vi "Execute Tests.vi"(8 "error in (no error)":errorcluster, 10 "Tests":string[](array[string]), 11 "Execution UI In":refnum<class "Execution UI.lvclass">) -> (0 "error out":errorcluster, 3 "Execution UI Out":refnum<class "Execution UI.lvclass">)   [LabVIEW 2020, in "Execution UI.lvclass"]
uses:
  Execution UI.lvclass
  TypeDefs/Execution State.ctl
  Result Model by Reference/Result Model by Reference.lvclass
  API/LUnit Test Suite/LUnit Test Suite.lvclass
  Support/Filters/Static Filter/Static Filter.lvclass
  Support/Filters/Dashed Filter/Dashed Filter.lvclass
  Support/Filters/Filter/Filter.lvclass
  Framework/Plugin/Plugin.lvclass
  Framework/Test Runner/Test Runner.lvclass
  C:/git/astemes-lunit/source/Core/Runnable/Runnable.lvclass
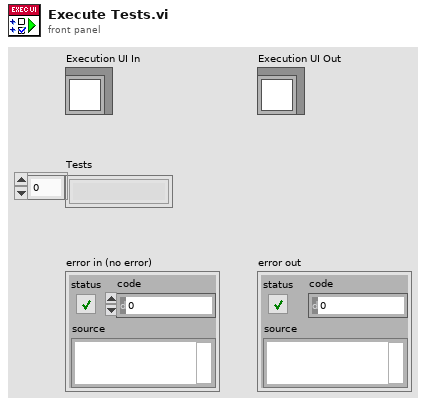
[diagram p1: front panel]
types:
  T1 = typedef "Execution UI.lvclass/Execution State.ctl" = enum16{"Idle", "Running"}
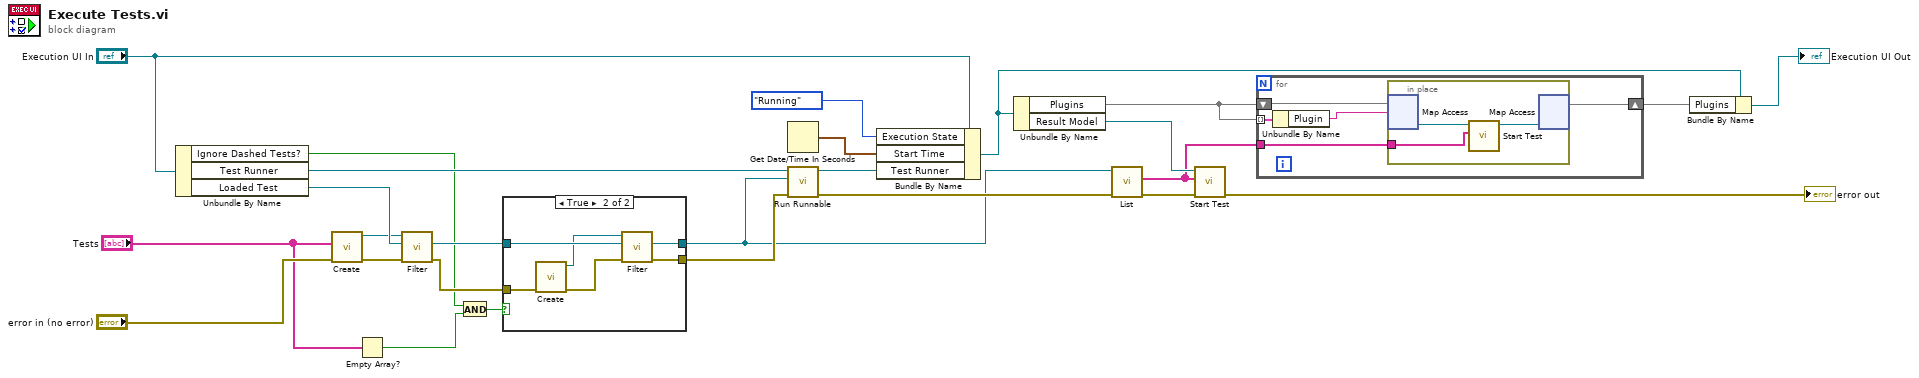
[diagram p0: block diagram]
diagram:
  n1 = Unbundle By Name("Execution UI In") -> ("Ignore Dashed Tests?"=w4:bool, "Test Runner"=w26:refnum<class "Test Runner.lvclass">, "Loaded Test"=w12:refnum<class "LUnit Test Suite.lvclass">)
  n2 = call "Create.vi"("error in (no error)"="error in (no error)", "Tests"="Tests") -> ("error out"=w9:errorcluster, "Static Filter"=w10:refnum<class "Filter.lvclass">)  [unwired: 8 in]
  n3 = Empty Array?(array="Tests") -> (empty?=w1:bool)
  n4 = call-dynamic "Filter.vi"("error in (no error)"=w9, "Test Suite"=w12, "Filter in"=w10) -> ("error out"=w7:errorcluster, "Filtered Test Suite"=w11:refnum<class "LUnit Test Suite.lvclass">)  [unwired: 7 in]
  n5 = And(x=w4, y=w1) -> (x .and. y?=w2:bool)
  n6 = case shown="True" w2 {
    tunnel: w7 -> [w27 w34]
    tunnel: [w27 w33] -> w6
    tunnel: w11 -> [w28 w32]
    tunnel: [w28 w31] -> w5
    frame False {
    }
    frame True {
      n7 = call "Create.vi"("error in (no error)"=w34) -> ("error out"=w30:errorcluster, "Dashed Filter"=w29:refnum<class "Dashed Filter.lvclass">)  [unwired: 9 in]
      n8 = call-dynamic "Filter.vi"("error in (no error)"=w30, "Test Suite"=w32, "Dashed Filter in"=w29) -> ("error out"=w33:errorcluster, "Filtered Test Suite"=w31:refnum<class "LUnit Test Suite.lvclass">)  [unwired: 7 in]
    }
  }
  n9 = Get Date/Time In Seconds() -> (seconds since 1Jan1904=w23:timestamp)
  n10 = call-dynamic "Run Runnable.vi"("error in (no error)"=w6, "Runnable"=w5, "Test Runner In"=w26) -> ("error out"=w15:errorcluster, "Test Runner Out"=w25:refnum<class "Test Runner.lvclass">)  [unwired: 7 in]
  n11 = Bundle By Name(cluster="Execution UI In", "Execution State"=Execution_State."Running", "Start Time"=w23, "Test Runner"=w25) -> (w17:refnum<class "Execution UI.lvclass">)
  n12 = Unbundle By Name(w17) -> ("Plugins"=w20:map{string, refnum<class "Plugin.lvclass">}, "Result Model"=w22:refnum<class "Result Model by Reference.lvclass">)
  n13 = call "List.vi"("error in (no error)"=w15, "LUnit Test Suite In"=w5) -> ("error out"=w14:errorcluster, "List of Runnables"=w13:string[])  [unwired: 8 in]
  n14 = call "Start Test.vi"("error in (no error)"=w14, "Tests"=w13, "Result Model In"=w22) -> ("error out"=→"error out":errorcluster)  [unwired: 8 in]
  n15 = for {
    tunnel: w13 -> [w36]
    shift-right: [w35] -> w21
    shift-left: w20 -> [w39]
    tunnel: w20 -> [w38] mode=indexing
    n16 = Unbundle By Name(w38) -> ("Plugin"=w37:string)
    n17 = in-place {
      in-place-border: w36 -> [w41]
      n18 = in-place-map #1(w39, w37) -> (w42:refnum<class "Plugin.lvclass">)  [unwired: 1 in, 1 out]
      n19 = call-dynamic "Start Test.vi"("Tests"=w41, "Plugin in"=w42) -> ("Plugin out"=w40:refnum<class "Plugin.lvclass">)  [unwired: 8 in, 1 out]
      n20 = in-place-map #1(w40) -> (w35:map{string, refnum<class "Plugin.lvclass">})  [unwired: 1 in, 2 out]
    }
  }
  n21 = Bundle By Name(cluster=w17, "Plugins"=w21) -> (→"Execution UI Out":refnum<class "Execution UI.lvclass">)
